vi "send_readID_commandv2.vi"() -> ()   [LabVIEW 2017]
panel:
  in  "数组 2":string[](array[string])=["shift:\u0005\u0000\u0000\u0000\u001f\u0000", "shift:\u0004\u0000\u0000\u0000\u0002\u0000", "shift: \u0000\u0000\u0000\u0000\u0000"]
  in  "数组 5":string[](array[string])=["shift:\u0006\u0000\u0000\u0000\u001f\u0000", "shift:\u0004\u0000\u0000\u0000\u0003\u0000", "shift:\u0006\u0000\u0000\u0000 ?", "shift:\u0002\u0000\u0000\u0000\u0001\u0000", "shift:\u0003\u0000\u0000\u0000\u0001\u0000", "shift:\b\u0000\u0000\u0000€¥", "shift:\u0002\u0000\u0000\u0000\u0001\u0000"]
  in  "shift string":string=":\u0005\u0000\u0000\u0000\u001f\u0000"
  out "number 2":u32=1 format="%x"
  out "number":u32=2 format="%x"
  out "数组 3":string[](array[string])=["", "", "", "", "_", "ÿ", "ÿ"]
  out "数据输出":string="ÿ"
  in  "数组":string[](array[string])=["shift:\u0005\u0000\u0000\u0000\u001f\u0000", "shift:\u0004\u0000\u0000\u0000\u0002\u0000", "shift: \u0000\u0000\u0000\u0000\u0000"]
  in  "服务器关闭":string="服务器VI关闭了连接。"
  in  "停止":bool
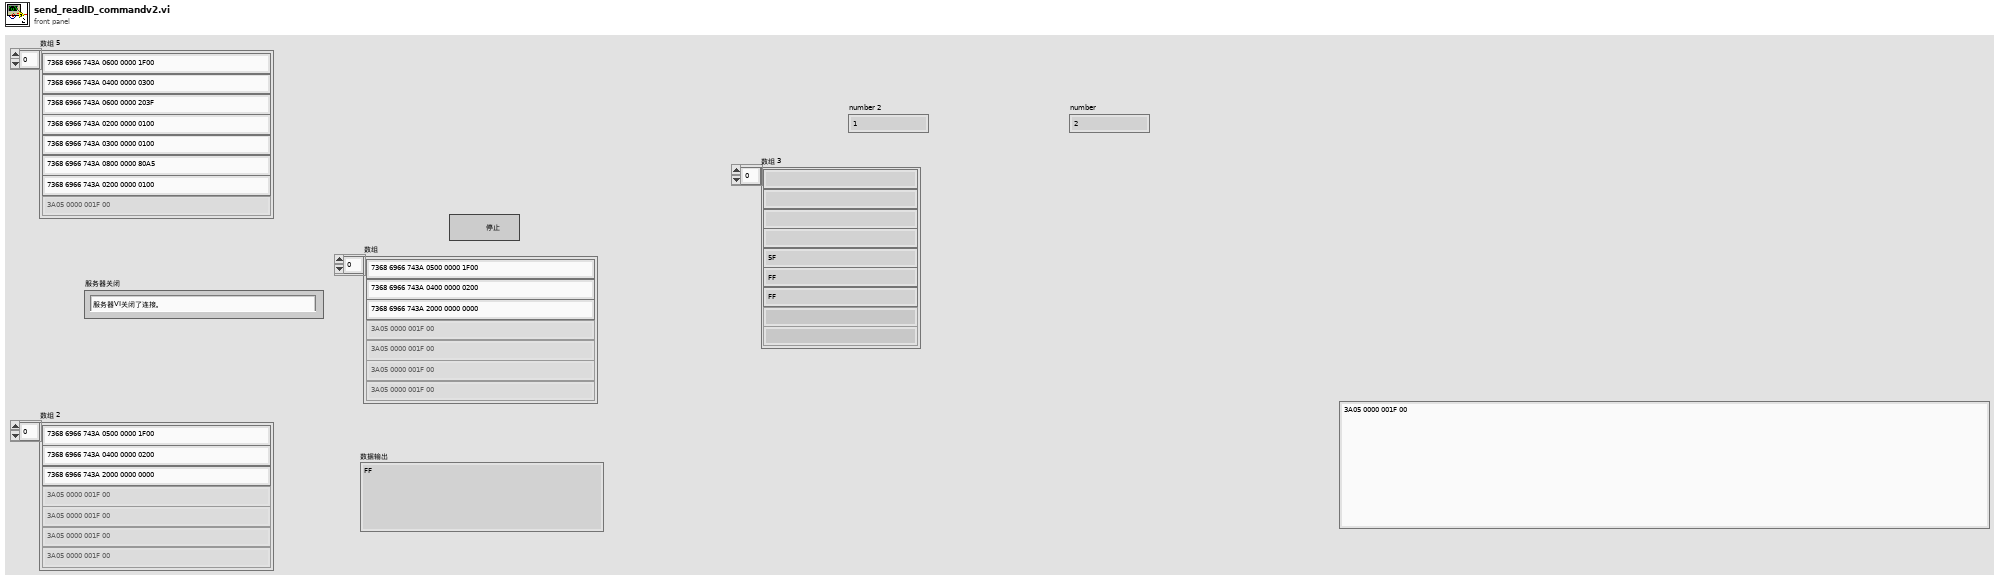
[diagram p1: front panel]
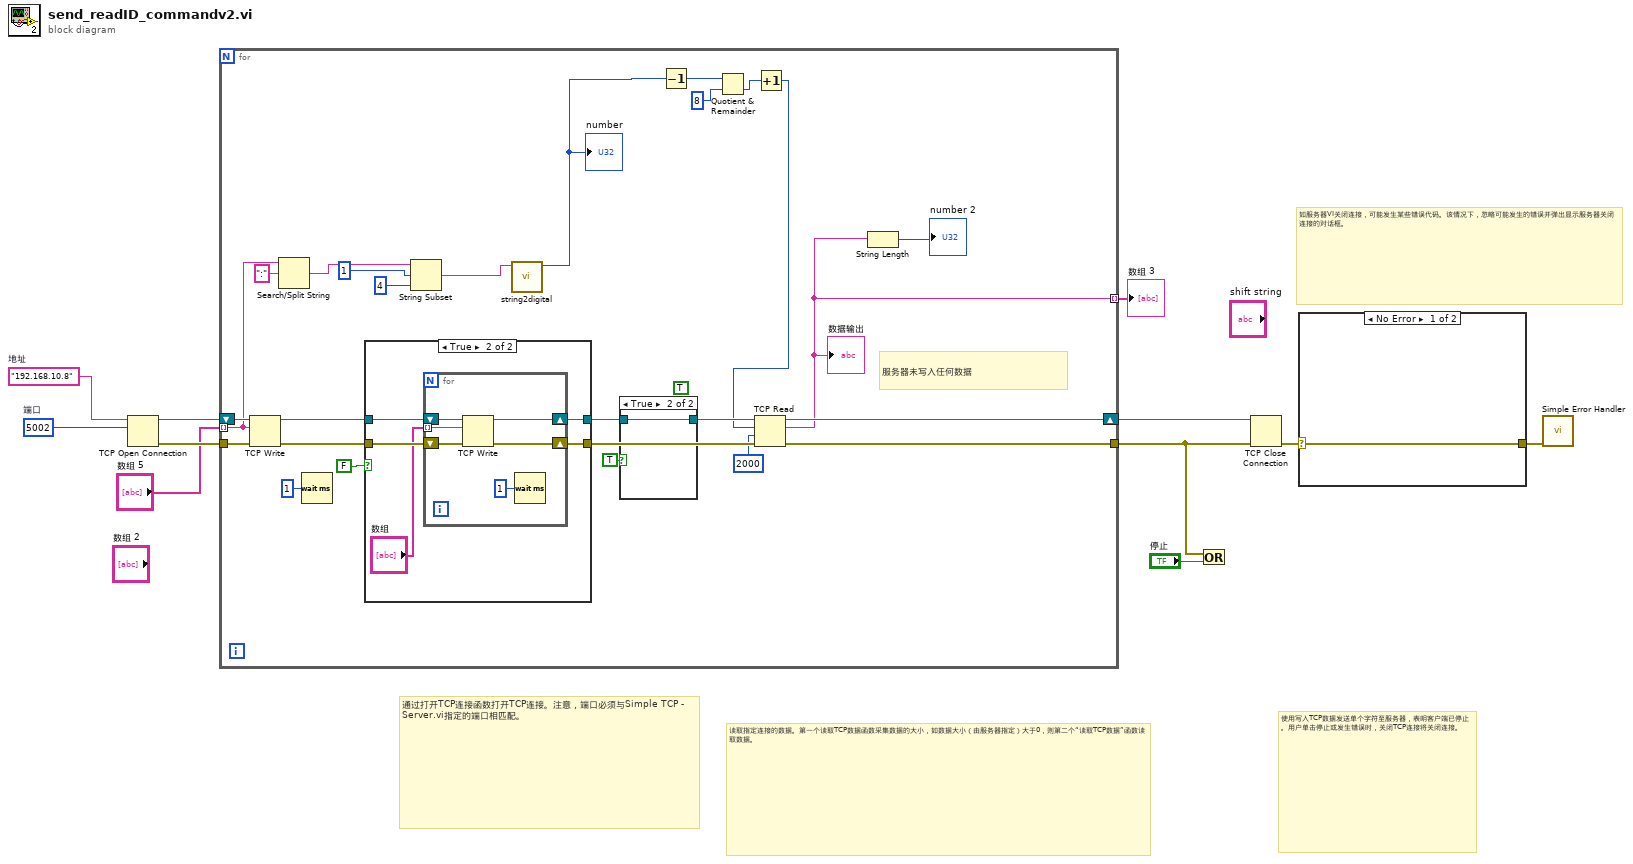
[diagram p0: block diagram]
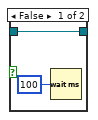
[diagram p2: hidden frame]
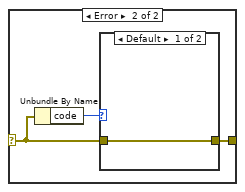
[diagram p4: hidden frame]
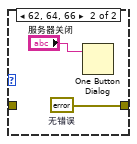
[diagram p5: hidden frame]
diagram:
  w8 = u16 5002  # 端口
  w9 = "192.168.10.8"  # 地址
  # "如服务器VI关闭连接，可能发生某些错误代码。该情况下，忽略可能发生的错误并弹出显示服务器关闭连接的对话框。"
  # "使用写入TCP数据发送单个字符至服务器，表明客户端已停止。用户单击停止或发生错误时，关闭TCP连接将关闭连接。"
  # "读取指定连接的数据。第一个读取TCP数据函数采集数据的大小，如数据大小（由服务器指定）大于0，则第二个“读取TCP数据”函数读取数据。"
  # "通过打开TCP连接函数打开TCP连接。注意，端口必须与Simple TCP - Server.vi指定的端口相匹配。"
  n1 = TCP Open Connection(address=w9, remote port or service name=w8) -> (connection ID=w7:refnum<k5>, error out=w6:errorcluster)  [unwired: 3 in]
  n2 = for {
    tunnel: "数组 5" -> [w15] mode=indexing
    shift-right: [w37] -> w3
    shift-left: w7 -> [w17]
    tunnel: [w13] -> w4 mode=indexing
    tunnel: w6 -> [w35]
    tunnel: [w36] -> w2
    (unwired) TRUE
    # "服务器未写入任何数据"
    n3 = TCP Write(connection ID=w17, data in=w15, error in (no error)=w35) -> (connection ID out=w34:refnum<k5>, error out=w33:errorcluster)  [unwired: 1 in, 1 out]
    n4 = Search/Split String(string=w15, search string/char (-)=":" ("正则表达式")) -> (match + rest of string=w16:string)  [unwired: 1 in, 2 out]
    n5 = Wait (ms)(milliseconds to wait=u32 1) -> ()  [unwired: 1 out]
    n6 = case shown="True" FALSE {
      tunnel: w34 -> [w42 w47]
      tunnel: w33 -> [w41 w46]
      tunnel: [w42 w45] -> w28
      tunnel: [w41 w44] -> w32
      frame False {
      }
      frame True {
        n7 = for {
          shift-right: [w51] -> w45
          shift-left: w47 -> [w53]
          shift-right: [w50] -> w44
          shift-left: w46 -> [w52]
          tunnel: "数组" -> [w49] mode=indexing
          n8 = TCP Write(connection ID=w53, data in=w49, error in (no error)=w52) -> (connection ID out=w51:refnum<k5>, error out=w50:errorcluster)  [unwired: 1 in, 1 out]
          n9 = Wait (ms)(milliseconds to wait=u32 1) -> ()  [unwired: 1 out]
        }
      }
    }
    n10 = String Subset(string=w16, offset (0)=1 ("length (rest)"), length (rest)=4 ("length (rest)")) -> (substring=w23:string)
    n11 = call "string2digital.vi"("data in"=w23) -> ("number"=w19:u32)  [unwired: 10 in]
    "number" <- w19
    n12 = case shown="True" TRUE {
      tunnel: w28 -> [w39 w40]
      tunnel: [w39 w40] -> w27
      frame False {
        n13 = Wait (ms)(milliseconds to wait=u32 100) -> ()  [unwired: 1 out]
      }
      frame True {
      }
    }
    n14 = Decrement(x=w19) -> (x-1=w21:u32)
    n15 = Quotient & Remainder(x=w21, y=u32 8) -> (floor(x/y)=w20:u32)  [unwired: 1 out]
    n16 = Increment(x=w20) -> (x+1=w14:u32)
    n17 = TCP Read(connection ID=w27, bytes to read=w14, error in (no error)=w32, 9:2000 ("timeout ms (25000)")) -> (connection ID out=w37:refnum<k5>, data out=w13:string, error out=w36:errorcluster)  [unwired: 1 in]
    "数据输出" <- w13
    n18 = String Length(string=w13) -> (length=→"number 2":i32)
  }
  "数组 3" <- w4
  n19 = Or(x=w2, y="停止") -> ()  [unwired: 1 out]
  n20 = TCP Close Connection(connection ID=w3, error in (no error)=w2) -> (error out=w11:errorcluster)  [unwired: 1 in, 1 out]
  n21 = case shown="No Error" w11 {
    selector: w11 -> [w54 w56]
    tunnel: [w54 w55] -> w10
    frame No Error {
    }
    frame Error {
      n22 = Unbundle By Name(w56) -> ("code"=w57:i32)
      n23 = case shown="Default" w57 {
        tunnel: w56 -> [w58 _]
        tunnel: [w58 w60] -> w55
        frame Default {
        }
        frame 62, 64, 66 {
          w60 = errorcluster {"status"=FALSE, "code"=0, "source"=""}  # 无错误
          n24 = One Button Dialog(message="服务器关闭") -> ()  [unwired: 1 in, 1 out]
        }
      }
    }
  }
  n25 = call <vilib>:"Simple Error Handler.vi"("error in (no error)"=w10) -> ()  [unwired: 4 in, 5 out]
